vi "20170418-lecture4-1 dynamic array.vi"() -> ()   [LabVIEW 2014]
panel:
  out "# of elements > 25":i32
  out "Array 2":dbl[](array[numeric])
  in  "# of elements":i32
  out "Array":dbl[](array[numeric])
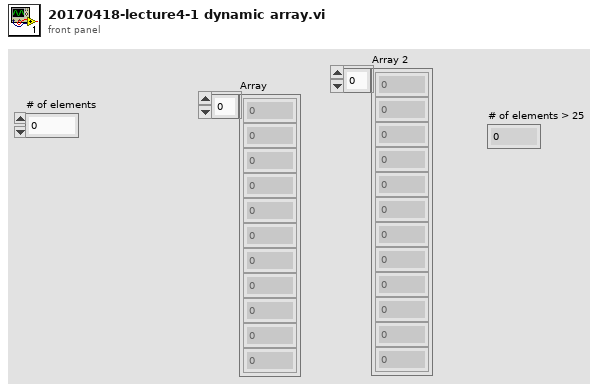
[diagram p1: front panel]
types:
  T1 = enum8{"Enabled", "Disabled", "Disabled and Grayed Out"}
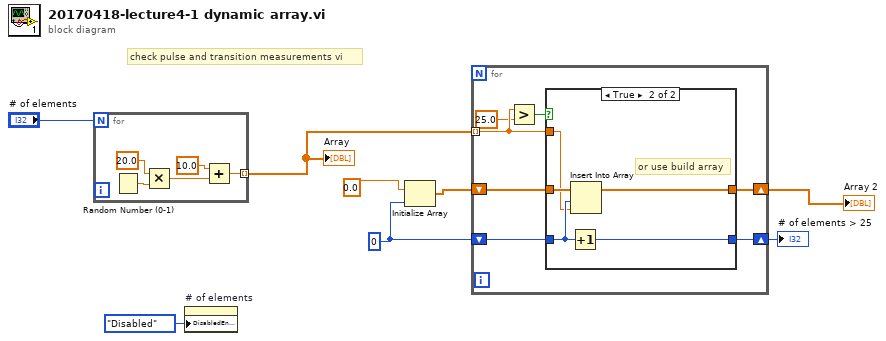
[diagram p0: block diagram]
diagram:
  w4 = 0 ("dimension size")
  # "check pulse and transition measurements vi"
  n1 = for {
    N: "# of elements" -> [_]
    tunnel: [w9] -> w5 mode=indexing
    n2 = Random Number (0-1)() -> (number: 0 to 1=w13:dbl)
    n3 = Multiply(x=20.0, y=w13) -> (x*y=w11:dbl)
    n4 = Add(x=10.0, y=w11) -> (x+y=w9:dbl)
  }
  "Array" <- w5
  n5 = property on="# of elements" class="DigNum (strict)"("DisabledEnum"=T1."Disabled" ("Disabled")) -> ()  [unwired: 2 in, 2 out]
  n6 = Initialize Array(0.0 ("element"), w4) -> (w7:dbl[])
  n7 = for {
    tunnel: w5 -> [w19] mode=indexing
    shift-right: [w17] -> w3
    shift-left: w7 -> [w18]
    shift-right: [w15] -> w2
    shift-left: w4 -> [w16]
    n8 = Greater?(x=w19, y=25.0) -> (0:w20:bool)
    n9 = case shown="True" w20 {
      tunnel: w19 -> [_ w23]
      tunnel: w18 -> [w22 w27]
      tunnel: [w22 w26] -> w17
      tunnel: w16 -> [w21 w25]
      tunnel: [w21 w24] -> w15
      frame False {
      }
      frame True {
        # "or use build array"
        n10 = Increment(x=w25) -> (x+1=w24:i32)
        n11 = Insert Into Array(array=w27, index=w25, new element=w23) -> (w26:dbl[])
      }
    }
  }
  "Array 2" <- w3
  "# of elements > 25" <- w2
